vi "SetParam.vi"(8 "error in (no error)":errorcluster caption="entrée d'erreur (pas d'erreur)", 10 "pairwise_distances":T1={"metric "="euclidean", "n_jobs"="None", "force_all_finite "="True"}, 11 "Pairwise_distances.lvclass":refnum<class "Pairwise_distances.lvclass">) -> (0 "error out":errorcluster caption="sortie d'erreur", 3 "Pairwise_distances.lvclass":refnum<class "Pairwise_distances.lvclass">)   [LabVIEW 2020, in "Pairwise_distances.lvclass"]
doc: "Set Parameters"
uses:
  Pairwise_distances.lvclass
  Pairwise_distances.lvclass/Pairwise_distances.ctl
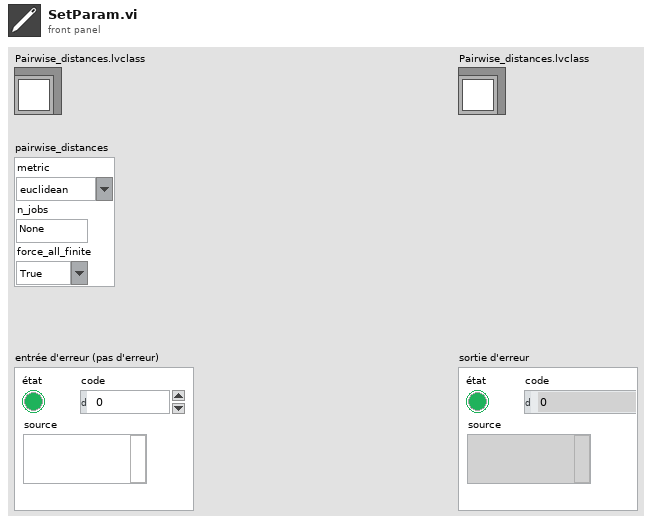
[diagram p1: front panel]
types:
  T1 = cluster{"metric ":string, "n_jobs":string, "force_all_finite ":string}
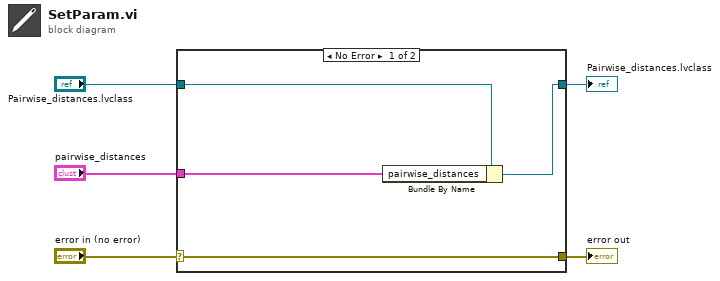
[diagram p0: block diagram]
diagram:
  n1 = case shown="No Error" "error in (no error)" {
    selector: "error in (no error)" -> [w9 w10]
    tunnel: [w9 w10] -> w4
    tunnel: [w7 w11] -> w2
    tunnel: "Pairwise_distances.lvclass" -> [w8 w11]
    tunnel: "pairwise_distances" -> [w6 _]
    frame No Error {
      n2 = Bundle By Name(cluster=w8, "pairwise_distances"=w6) -> (w7:refnum<class "Pairwise_distances.lvclass">)
    }
    frame Error {
    }
  }
  "error out" <- w4
  "Pairwise_distances.lvclass" <- w2
